vi "ADO Connection Create Table.vi"(6 "primary key (-1)":i32=-1, 7 "file?":bool, 8 "error in (no error)":errorcluster caption="错误输入（无错误）", 9 "column information":T2(array[cluster]), 10 "table":string, 11 "Database Connection.lvclass In":refnum<class "Database Connection.lvclass">) -> (0 "error IO":errorcluster, 3 "Database Connection.lvclass Out":refnum<class "Database Connection.lvclass">)   [LabVIEW 2011, in "Database Connection.lvclass"]
uses:
  Database Connection.lvclass
  <vilib>/addons/database/Auxilliary.llb/DB Tools DataTypes.ctl
  Recordset/Database Recordset.lvclass
  <vilib>/addons/database/NI_Database_API.lvlib
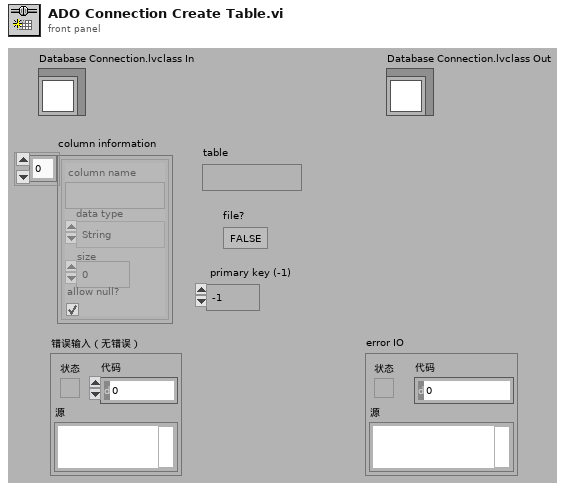
[diagram p1: front panel]
types:
  T1 = typedef "NI_Database_API.lvlib/DB Tools DataTypes.ctl" = enum16{"String", "Long (I32)", "Single (SGL)", "Double (DBL)", "Date/Time", "Binary"}
  T2 = cluster{"column name":string, "data type":T1, "size":i32, "allow null?":bool}[]
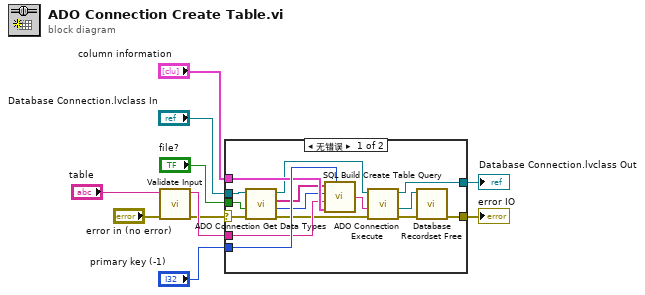
[diagram p0: block diagram]
diagram:
  n1 = call "Validate Input.vi"("error in (no error)"="error in (no error)", "table"="table") -> ("error out"=w7:errorcluster, "table out"=w8:string)  [unwired: 7 in, 1 out]
  n2 = case shown="无错误" w7 {
    selector: w7 -> [w22 w27]
    tunnel: w8 -> [w18 _]
    tunnel: [w12 w27] -> w4
    tunnel: "primary key (-1)" -> [w25 _]
    tunnel: "column information" -> [w24 _]
    tunnel: "file?" -> [w23 _]
    tunnel: "Database Connection.lvclass In" -> [w21 w26]
    tunnel: [w14 w26] -> w2
    frame No Error {
      n3 = call "ADO Connection Get Data Types.vi"("error in (no error)"=w22, "file?"=w23, "Database Connection 输入"=w21) -> ("error out"=w15:errorcluster, "database"=w19:enum16{"dBase", "Jet", "SQL Server", "Oracle"}, "data types"=w20:string[], "Database Connection 输出"=w16:refnum<class "Database Connection.lvclass">)  [unwired: 5 in]
      n4 = call "SQL Build Create Table Query.vi"("data types"=w20, "database"=w19, "table"=w18, "column information"=w24, "primary key (-1)"=w25) -> ("字符串"=w17:string)
      n5 = call "ADO Connection Execute.vi"("error in (no error)"=w15, "CommandText"=w17, "Database Connection 输入"=w16) -> ("error out"=w13:errorcluster, "Database Recordset输出"=w11:refnum<class "Database Recordset.lvclass">, "Database Connection 输出"=w14:refnum<class "Database Connection.lvclass">)  [unwired: 6 in]
      n6 = call "Database Recordset Free.vi"("error in (no error)"=w13, "Database Recordset 输入"=w11) -> ("error out"=w12:errorcluster)  [unwired: 9 in]
    }
    frame Error {
    }
  }
  "Database Connection.lvclass Out" <- w2
  "error IO" <- w4
